vi "Get Palette Menu Information.vi"() -> ()   [LabVIEW 2022 SP3]
uses:
  System.Drawing
panel:
  out "Array":T1(array[cluster])
  in  "Palette Menu Path":path
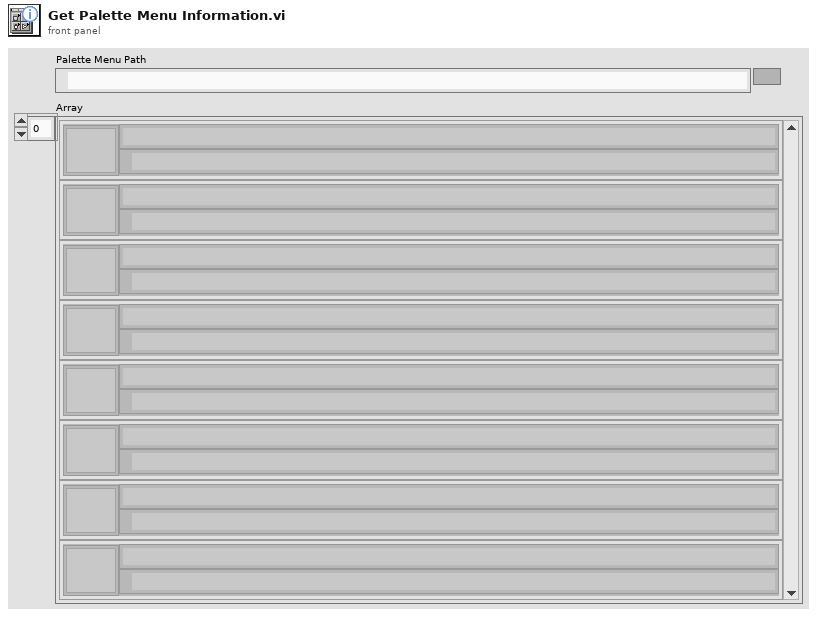
[diagram p1: front panel]
types:
  T1 = cluster{"Name":string, "Path":path, "Icon":picture}[]
  T2 = cluster{"Palette Item Type":enum32{"Submenu", "VI", "Express VI", "Built In", "Empty"}, "short name":string, "Item name":string, "file path":path, "image":u8[]}[]
  T3 = cluster{"Item name":string, "file path":path, "new picture":picture}
  T4 = typedef "imagedata.ctl" = cluster{"image type":i32, "image depth":i32, "image":u8[], "mask":u8[], "colors":u32[], "Rectangle":cluster{"left":i16, "top":i16, "right":i16, "bottom":i16}}
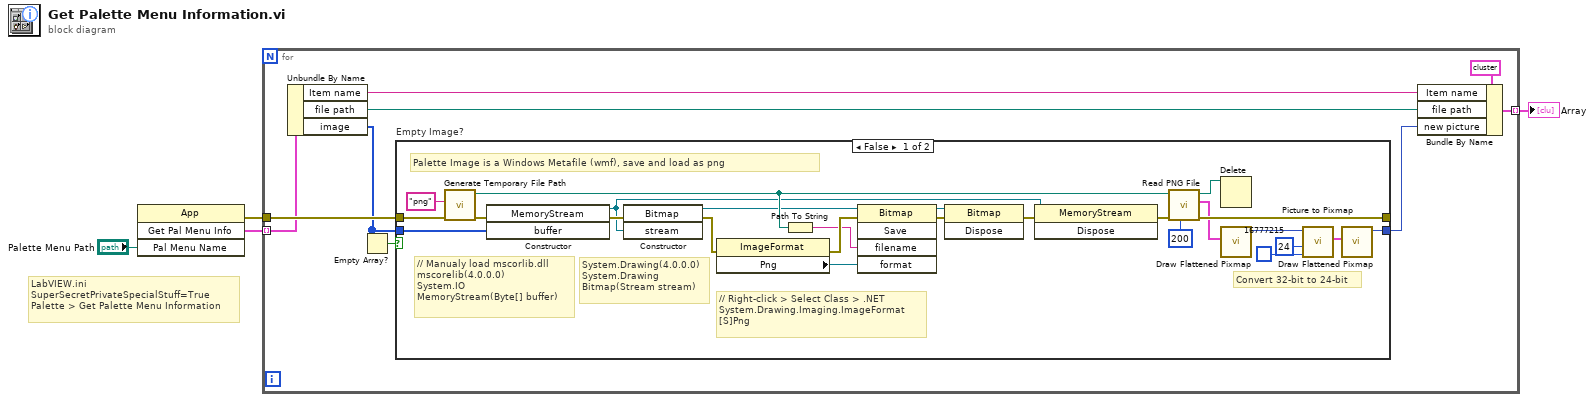
[diagram p0: block diagram]
diagram:
  # "LabVIEW.ini\nSuperSecretPrivateSpecialStuff=True\nPalette > Get Palette Menu Information"
  n1 = invoke class="App" method="Get Pal Menu Info"("Pal Menu Name"="Palette Menu Path") -> (error out=w4:errorcluster, "Get Palette Menu Info"=w3:T2)  [unwired: 3 in, 2 out]
  n2 = for {
    tunnel: w4 -> [w12]
    tunnel: w3 -> [w11] mode=indexing
    tunnel: [w5] -> w1 mode=indexing
    n3 = Unbundle By Name(w11) -> ("Item name"=w9:string, "file path"=w8:path, "image"=w10:u8[])
    n4 = Empty Array?(array=w10) -> (empty?=w13:bool)
    n5 = case "Empty Image?" shown="False" w13 {
      tunnel: w10 -> [w38 _]
      tunnel: [w31 w39] -> _
      tunnel: w12 -> [w30 w39]
      tunnel: [w14 _] -> w7
      frame False {
        # "Convert 32-bit to 24-bit"
        # "Palette Image is a Windows Metafile (wmf), save and load as png"
        # "// Right-click > Select Class > .NET\nSystem.Drawing.Imaging.ImageFormat\n[S]Png"
        # "System.Drawing(4.0.0.0)\nSystem.Drawing\nBitmap(Stream stream)"
        # "// Manualy load mscorlib.dll\nmscorelib(4.0.0.0)\nSystem.IO\nMemoryStream(Byte[] buffer)"
        n6 = call <vilib>:"Generate Temporary File Path.vi"("error in (no error)"=w30, "Temporary File Extension (tmp)"="png") -> ("error out"=w29:errorcluster, "Unique Temporary File Path"=w27:path)  [unwired: 8 in]
        n7 = constructor class="MemoryStream"(error in=w29, "buffer"=w38) -> (reference out=w21:refnum<k24>, error out=w37:errorcluster)  [unwired: 2 in, 2 out]
        n8 = constructor class="Bitmap"(error in=w37, "stream"=w21) -> (reference out=w16:refnum<k24>, error out=w34:errorcluster)  [unwired: 2 in, 2 out]
        n9 = property class="ImageFormat"(error in=w34) -> (error out=w33:errorcluster, "Png"=w25:refnum<k24>)  [unwired: 1 in, 1 out]
        n10 = Path To String(path=w27) -> (string=w20:string)
        n11 = invoke class="Bitmap" method="Save"(reference=w16, error in=w33, "filename"=w20, "format"=w25) -> (reference out=w36:refnum<k24>, error out=w35:errorcluster)  [unwired: 1 in, 3 out]
        n12 = invoke class="Bitmap" method="Dispose"(reference=w36, error in=w35) -> (error out=w19:errorcluster)  [unwired: 1 in, 2 out]
        n13 = invoke class="MemoryStream" method="Dispose"(reference=w21, error in=w19) -> (error out=w32:errorcluster)  [unwired: 1 in, 2 out]
        n14 = call <vilib>:"Read PNG File.vi"("Transparency Thresh"=u8 200, "error in (no error)"=w32, "path to PNG file"=w27) -> ("error out"=w31:errorcluster, "image data"=w17:T4, "path"=w26:path)  [unwired: 6 in]
        n15 = Delete(path (use dialog)=w26) -> ()  [unwired: 4 in, 3 out]
        n16 = call <vilib>:"Draw Flattened Pixmap.vi"("image data"=w17) -> ("new picture"=w24:picture)  [unwired: 8 in]
        n17 = call <vilib>:"Picture to Pixmap.vi"("Background Color"=u32 16777215, "depth"=24, "picture"=w24) -> ("image data"=w15:T4)  [unwired: 7 in, 1 out]
        n18 = call <vilib>:"Draw Flattened Pixmap.vi"("image data"=w15) -> ("new picture"=w14:picture)  [unwired: 8 in]
      }
      frame True {
      }
    }
    n19 = Bundle By Name(cluster=T3 {"Item name"="", "file path"=path "", "new picture"=bytes[0]}, "Item name"=w9, "file path"=w8, "new picture"=w7) -> (w5:T3)
  }
  "Array" <- w1
